vi "4_8.vi"() -> ()   [LabVIEW 2020]
panel:
  out "Output":string
  in  "Input":string
  out "String 2":string
  out "unsigned byte array":u8[](array[numeric])
  in  "String":string
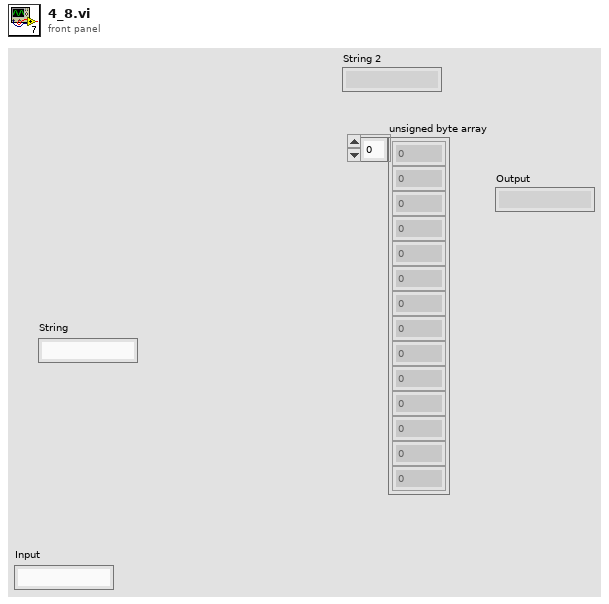
[diagram p1: front panel]
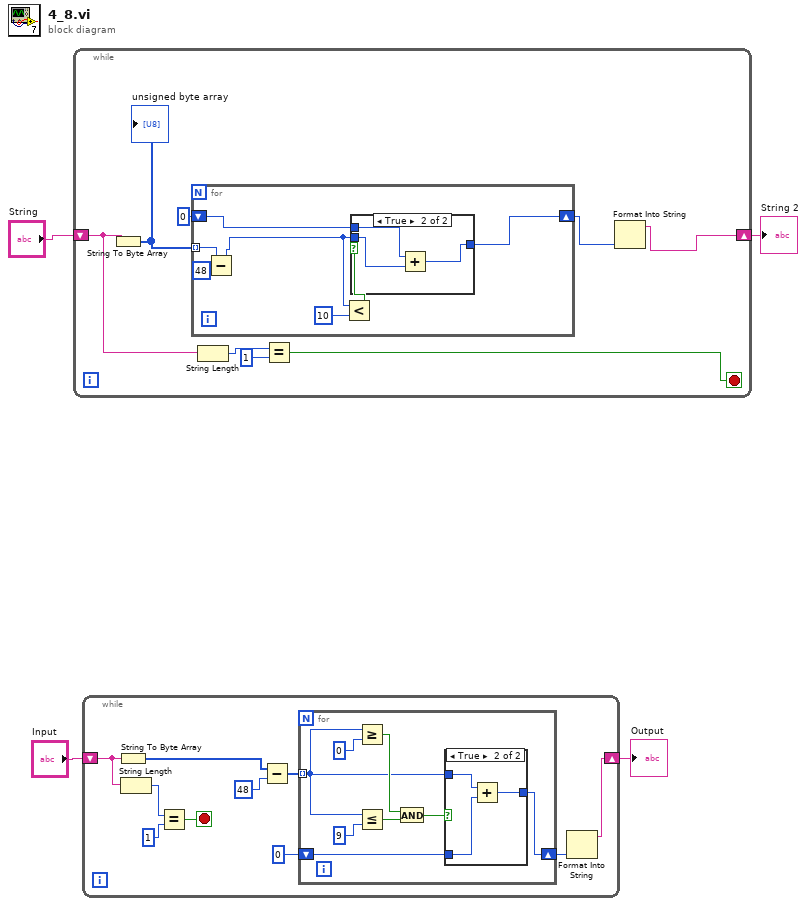
[diagram p0: block diagram]
diagram:
  n1 = while {
    shift-right: [w8] -> w3
    shift-left: "String" -> [w9]
    stop <- w5 stop-if-true
    n2 = String To Byte Array(string=w9) -> (unsigned byte array=w12:u8[])
    "unsigned byte array" <- w12
    n3 = for {
      tunnel: w12 -> [w16] mode=indexing
      shift-right: [w19] -> w10
      shift-left: u8 0 -> [w18]
      n4 = Subtract(x=w16, y=u8 48) -> (x-y=w13:u8)
      n5 = Less?(x=w13, y=u8 10) -> (x < y?=w15:bool)
      n6 = case shown="True" w15 {
        tunnel: [w20 w21] -> w19
        tunnel: w13 -> [_ w22]
        tunnel: w18 -> [w20 w23]
        frame False {
        }
        frame True {
          n7 = Add(x=w23, y=w22) -> (x+y=w21:u8)
        }
      }
    }
    n8 = String Length(string=w9) -> (length=w7:i32)
    n9 = Equal?(x=w7, y=1) -> (x = y?=w5:bool)
    n10 = Format Into String(w10) -> (resulting string=w8:string)  [unwired: 3 in, 1 out]
  }
  "String 2" <- w3
  n11 = while {
    shift-right: [w28] -> w1
    shift-left: "Input" -> [w27]
    stop <- w24 stop-if-true
    n12 = String To Byte Array(string=w27) -> (unsigned byte array=w33:u8[])
    n13 = String Length(string=w27) -> (length=w26:i32)
    n14 = Equal?(x=w26, y=1) -> (x = y?=w24:bool)
    n15 = Subtract(x=w33, y=48) -> (x-y=w31:i32[])
    n16 = for {
      tunnel: w31 -> [w36] mode=indexing
      shift-right: [w34] -> w29
      shift-left: 0 -> [w35]
      n17 = Greater Or Equal?(x=w36, y=0) -> (x >= y?=w38:bool)
      n18 = Less Or Equal?(x=w36, y=9) -> (x <= y?=w37:bool)
      n19 = And(x=w38, y=w37) -> (x .and. y?=w41:bool)
      n20 = case shown="True" w41 {
        tunnel: w36 -> [_ w45]
        tunnel: w35 -> [w42 w44]
        tunnel: [w42 w43] -> w34
        frame False {
        }
        frame True {
          n21 = Add(x=w45, y=w44) -> (x+y=w43:i32)
        }
      }
    }
    n22 = Format Into String(w29) -> (resulting string=w28:string)  [unwired: 3 in, 1 out]
  }
  "Output" <- w1
